vi "fit mag to ellipse with more parameters.vi"(7 "advanced fit":bool, 8 "starting parameters":dbl[](array[numeric]), 9 "T":dbl, 10 "t0":dbl, 11 "mag no drive":T2[](array[typedef])) -> (1 "fitter error":bool, 2 "fit magnetic field":T2[](array[typedef]), 3 "fit parameters":T1)   [LabVIEW 2017]
uses:
  typedefs/reading.ctl
  typedefs/readingType.ctl
  typedefs/magnetic field fit.ctl
  <vilib>/Analysis/baseanly.llb/Mean (DBL).vi
  <vilib>/gmath/NumericalOptimization/Nonlinear Curve Fit LM bound.vi
  <vilib>/gmath/NI_Gmath.lvlib
  <vilib>/Analysis/NI_AALBase.lvlib
panel:
  out "number of function calls":i32
  out "residue":dbl
  out "phi":dbl[](array[numeric])
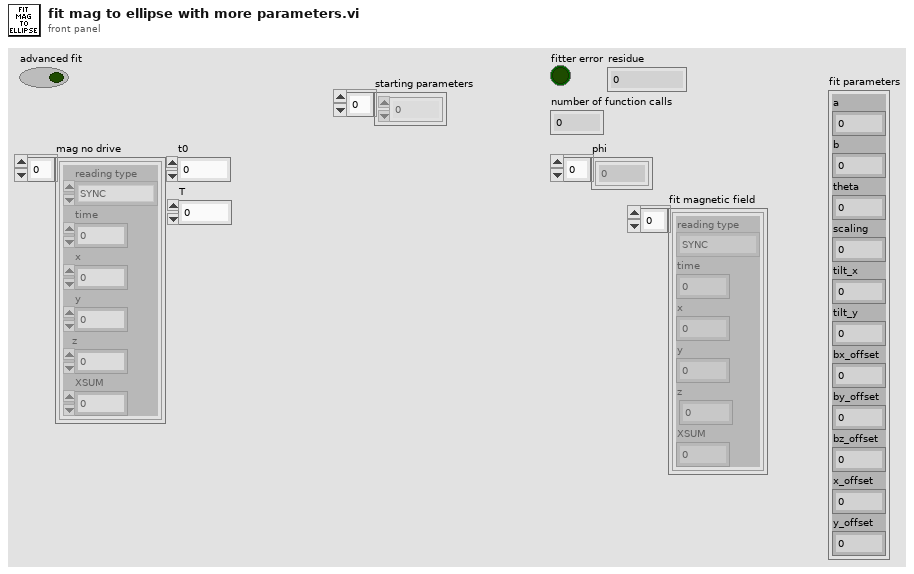
[diagram p1: front panel]
types:
  T1 = typedef "magnetic field fit.ctl" = cluster{"a":dbl, "b":dbl, "theta":dbl, "scaling":dbl, "tilt_x":dbl, "tilt_y":dbl, "bx_offset":dbl, "by_offset":dbl, "bz_offset":dbl, "x_offset":dbl, "y_offset":dbl}
  T2 = typedef "reading.ctl" = cluster{"reading type":T3, "time":fxp<+,48,48>, "x":sgl, "y":sgl, "z":sgl, "XSUM":u8}
  T3 = typedef "readingType.ctl" = enum8{"SYNC", "DETVAL", "COILI", "MAGVEC", "ACCVEC"}
  T4 = cluster{"best fit parameters[0]":dbl, "best fit parameters[1]":dbl, "best fit parameters[2]":dbl, "best fit parameters[3]":dbl, "best fit parameters[4]":dbl, "best fit parameters[5]":dbl, "best fit parameters[6]":dbl, "best fit parameters[7]":dbl, "best fit parameters[8]":dbl, "best fit parameters[9]":dbl, "best fit parameters[10]":dbl}
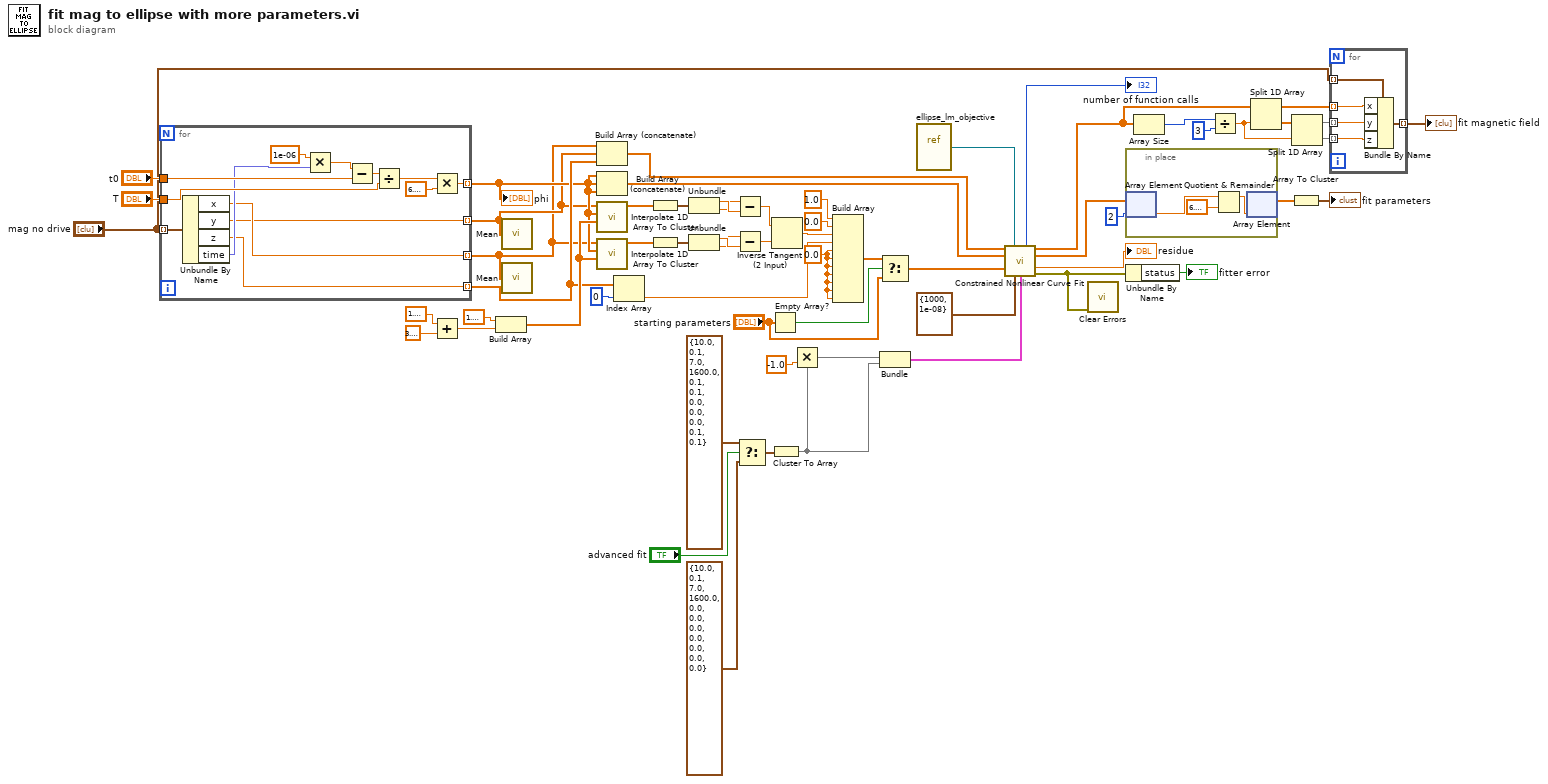
[diagram p0: block diagram]
diagram:
  w9 = 0.0
  n1 = for {
    tunnel: "mag no drive" -> [w74] mode=indexing
    tunnel: "T" -> [w71]
    tunnel: "t0" -> [w73]
    tunnel: [w65] -> w27 mode=indexing
    tunnel: [w64] -> w10 mode=indexing
    tunnel: [w63] -> w11 mode=indexing
    tunnel: [w62] -> w39 mode=indexing
    n2 = Unbundle By Name(w74) -> ("x"=w64:sgl, "y"=w63:sgl, "z"=w62:sgl, "time"=w68:fxp<+,48,48>)
    n3 = Multiply(x=1e-06, y=w68) -> (x*y=w67:dbl)
    n4 = Subtract(x=w67, y=w73) -> (x-y=w72:dbl)
    n5 = Divide(x=w72, y=w71) -> (x/y=w70:dbl)
    n6 = Multiply(x=w70, y=6.283185307179586) -> (x*y=w65:dbl)
  }
  "phi" <- w27
  n7 = Add(x=1.5707963267948966, y=3.141592653589793) -> (x+y=w56:dbl)
  n8 = Build Array(1.5707963267948966, w56) -> (w55:dbl[])
  n9 = call-poly <vilib>:"Mean.vi"("X"=w11) -> ()  [unwired: 2 out]
  n10 = call-poly <vilib>:"Mean.vi"("X"=w10) -> ()  [unwired: 2 out]
  n11 = Build Array (concatenate)(w10, w11, w39) -> (w38:sgl[])
  n12 = Build Array (concatenate)(w27, w27, w27) -> (w28:dbl[])
  n13 = call <vilib>:"Interpolate 1D.vi"("xi"=w55, "X"=w27, "Y"=w11) -> ("yi"=w53:dbl[])  [unwired: 6 in, 2 out]
  n14 = call <vilib>:"Interpolate 1D.vi"("xi"=w55, "X"=w27, "Y"=w10) -> ("yi"=w54:dbl[])  [unwired: 6 in, 2 out]
  n15 = Index Array(array=w39, index=0) -> (element=w40:sgl)
  n16 = Array To Cluster(array=w53) -> (cluster=w51:cluster{"yi[0]":dbl, "yi[1]":dbl})
  n17 = Array To Cluster(array=w54) -> (cluster=w52:cluster{"yi[0]":dbl, "yi[1]":dbl})
  n18 = Unbundle(w51) -> ("yi[0]"=w48:dbl, "yi[1]"=w47:dbl)
  n19 = Unbundle(w52) -> ("yi[0]"=w50:dbl, "yi[1]"=w49:dbl)
  n20 = Subtract(x=w47, y=w48) -> (x-y=w46:dbl)
  n21 = Subtract(x=w49, y=w50) -> (x-y=w45:dbl)
  n22 = Select(t=T1 {"a"=10.0, "b"=0.1, "theta"=7.0, "scaling"=1600.0, "tilt_x"=0.1, "tilt_y"=0.1, "bx_offset"=0.0, "by_offset"=0.0, "bz_offset"=0.0, "x_offset"=0.1, "y_offset"=0.1} ("fit parameters 2"), s="advanced fit", f=T1 {"a"=10.0, "b"=0.1, "theta"=7.0, "scaling"=1600.0, "tilt_x"=0.0, "tilt_y"=0.0, "bx_offset"=0.0, "by_offset"=0.0, "bz_offset"=0.0, "x_offset"=0.0, "y_offset"=0.0} ("fit parameters 2")) -> (s? t:f=w2:T1)
  n23 = Empty Array?(array="starting parameters") -> (empty?=w21:bool)
  n24 = Cluster To Array(cluster=w2) -> (array=w16:dbl[])
  n25 = Inverse Tangent (2 Input)(1:w45, 2:w46) -> (0:w41:dbl)
  n26 = Multiply(x=w16, y=-1.0) -> (x*y=w1:dbl[])
  n27 = Build Array(1.0 ("element"), 0.0 ("element"), w41, w40, w9, w9, w9, w9, w9, w9, w9) -> (w23:dbl[])
  n28 = Select(t=w23, s=w21, f="starting parameters") -> (s? t:f=w22:dbl[])
  n29 = Bundle(w1, "fit parameters 2"=w16) -> (w15:cluster{dbl[], "fit parameters 2":dbl[]})  [unwired: 1 in]
  n30 = vi-ref "ellipse_lm_objective.vi"() -> (w37:refnum<vi>)
  n31 = call-poly <vilib>:"Constrained Nonlinear Curve Fit.vi"("Y"=w38, "f(x,a)"=w37, "X"=w28, "initial parameters"=w22, "termination"=cluster{"max iteration":i32, "tolerance":dbl} {"max iteration"=1000, "tolerance"=1e-08}, "parameter bounds"=w15) -> ("number of function calls"=→"number of function calls":i32, "best nonlinear fit"=w26:dbl[], "best fit parameters"=w14:dbl[], "residue"=→"residue":dbl, "error out"=w29:errorcluster)  [unwired: 4 in, 1 out]
  n32 = call <vilib>:"Clear Errors.vi"("error in (no error)"=w29) -> ()  [unwired: 5 in, 2 out]
  n33 = in-place {
    n34 = in-place-array #1(w14, 2) -> (w77:dbl)
    n35 = Quotient & Remainder(x=w77, y=6.283185307179586) -> (x-y*floor(x/y)=w75:dbl)  [unwired: 1 out]
    n36 = in-place-array #1(w75) -> (w12:dbl[])  [unwired: 1 out]
  }
  n37 = Unbundle By Name(w29) -> ("status"=→"fitter error":bool)
  n38 = Array Size(array=w26) -> (size(s)=w36:i32)
  n39 = Divide(x=w36, y=3) -> (x/y=w24:dbl)
  n40 = Split 1D Array(array=w26, index=w24) -> (first subarray=w34:dbl[], second subarray=w25:dbl[])
  n41 = Array To Cluster(array=w12) -> (cluster=→"fit parameters":T4)
  n42 = Split 1D Array(array=w25, index=w24) -> (first subarray=w33:dbl[], second subarray=w32:dbl[])
  n43 = for {
    tunnel: w34 -> [w81] mode=indexing
    tunnel: w33 -> [w80] mode=indexing
    tunnel: w32 -> [w79] mode=indexing
    tunnel: "mag no drive" -> [w82] mode=indexing
    tunnel: [w78] -> w30 mode=indexing
    n44 = Bundle By Name(cluster=w82, "x"=w81, "y"=w80, "z"=w79) -> (w78:T2)
  }
  "fit magnetic field" <- w30
